vi "Relay Experiment V2 - Curves.vi"() -> ()   [LabVIEW 2020]
uses:
  <vilib>/Analysis/8numeric.llb/1D Numeric Integration.vi
  <vilib>/DAQmx/write.llb/DAQmx Write (Analog 1D Wfm NChan NSamp).vi
  <vilib>/DAQmx/create/channels.llb/DAQmx Create Channel (AO-Voltage-Basic).vi
  <vilib>/DAQmx/configure/timing.llb/DAQmx Timing (Use Waveform).vi
  <vilib>/DAQmx/miscellaneous.llb/DAQmx Fill In Error Info.vi
  <vilib>/Analysis/NI_AALBase.lvlib
  <vilib>/measure/NI_MABase.lvlib
  <vilib>/Analysis/NI_AALPro.lvlib
panel:
  in  "Test Mode?":bool
  out "Charge (mC)":dbl
  in  "Recharge\nAmplitude (mA)":dbl=0.1
  in  "DC-to-AC \nDelay (ms)":dbl
  in  "Pulse\nAmplitude (mA)":dbl=-5.0
  in  "Pulse Plateau\nTime (ms) (g)":dbl=5000.0
  in  "Post-Pulse-\nSecond Curve (j)\nRadius (ms/mA)":dbl=150.0
  in  "Post-Pulse - \nFirst Curve (i)\nRadius (ms/mA)":dbl=50.0
  in  "Post-Pulse Curve \nTotal Time (ms) (h)":dbl=750.0
  in  "Recharge-Pulse -\nSecond Curve (f)\nRadius (ms/mA)":dbl=100.0
  in  "Recharge-Pulse - \nFirst Curve (e)\nRadius (ms/mA)":dbl=2000.0
  in  "Recharge-Pulse Curve\nTotal Time (ms) (d)":dbl=2100.0
  in  "Pre-Recharge -\nSecond Curve (c)\nRadius (ms/mA)":dbl=10000.0
  in  "Pre-Recharge -  \nFirst Curve (b)\nRadius (ms/mA)":dbl=10000.0
  in  "Pre-Recharge\nCurve Total\nTime (ms) (a)":dbl=2000.0
  in  "Trigger 2 Channel":tag="Dev2/ao3"
  in  "AC Output Channel":tag="Dev2/ao1"
  in  "Trigger 1 Channel":tag="Dev2/ao2"
  in  "DC Output Channel":tag="Dev2/ao0"
  in  "Stop":bool
  in  "AC Source\nGain":dbl=5.0
  out "DC On":bool=TRUE
  out "AC On":bool
  in  "Waveform Type":u16(ring) items=["Sine Wave", "Triangle Wave", "Square Wave", "Sawtooth Wave"]
  out "DC Waveform Graph":waveform(dbl)(graph)
  in  "AC  Waveform\nFrequency (Hz)":i32=20000 min=0 max=100000 step=10
  in  "AC  Waveform\nAmplitude\n(Vpp/mApp)":dbl
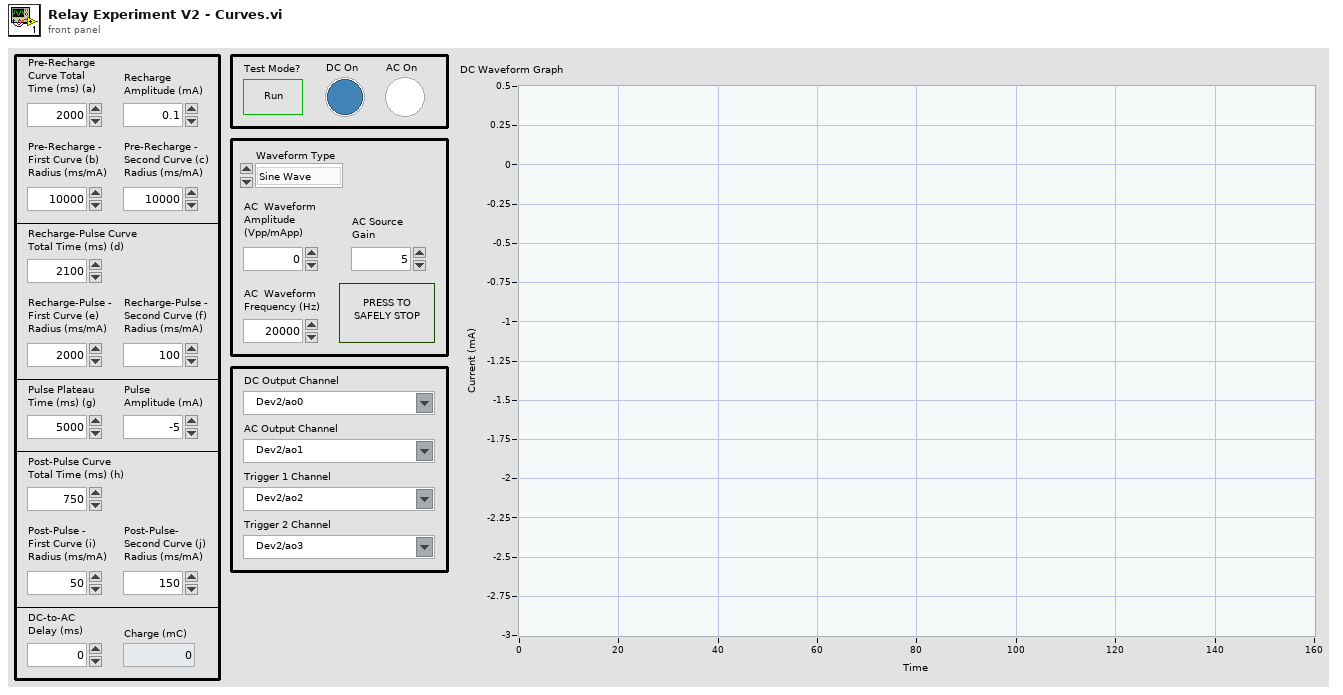
[diagram p1: front panel]
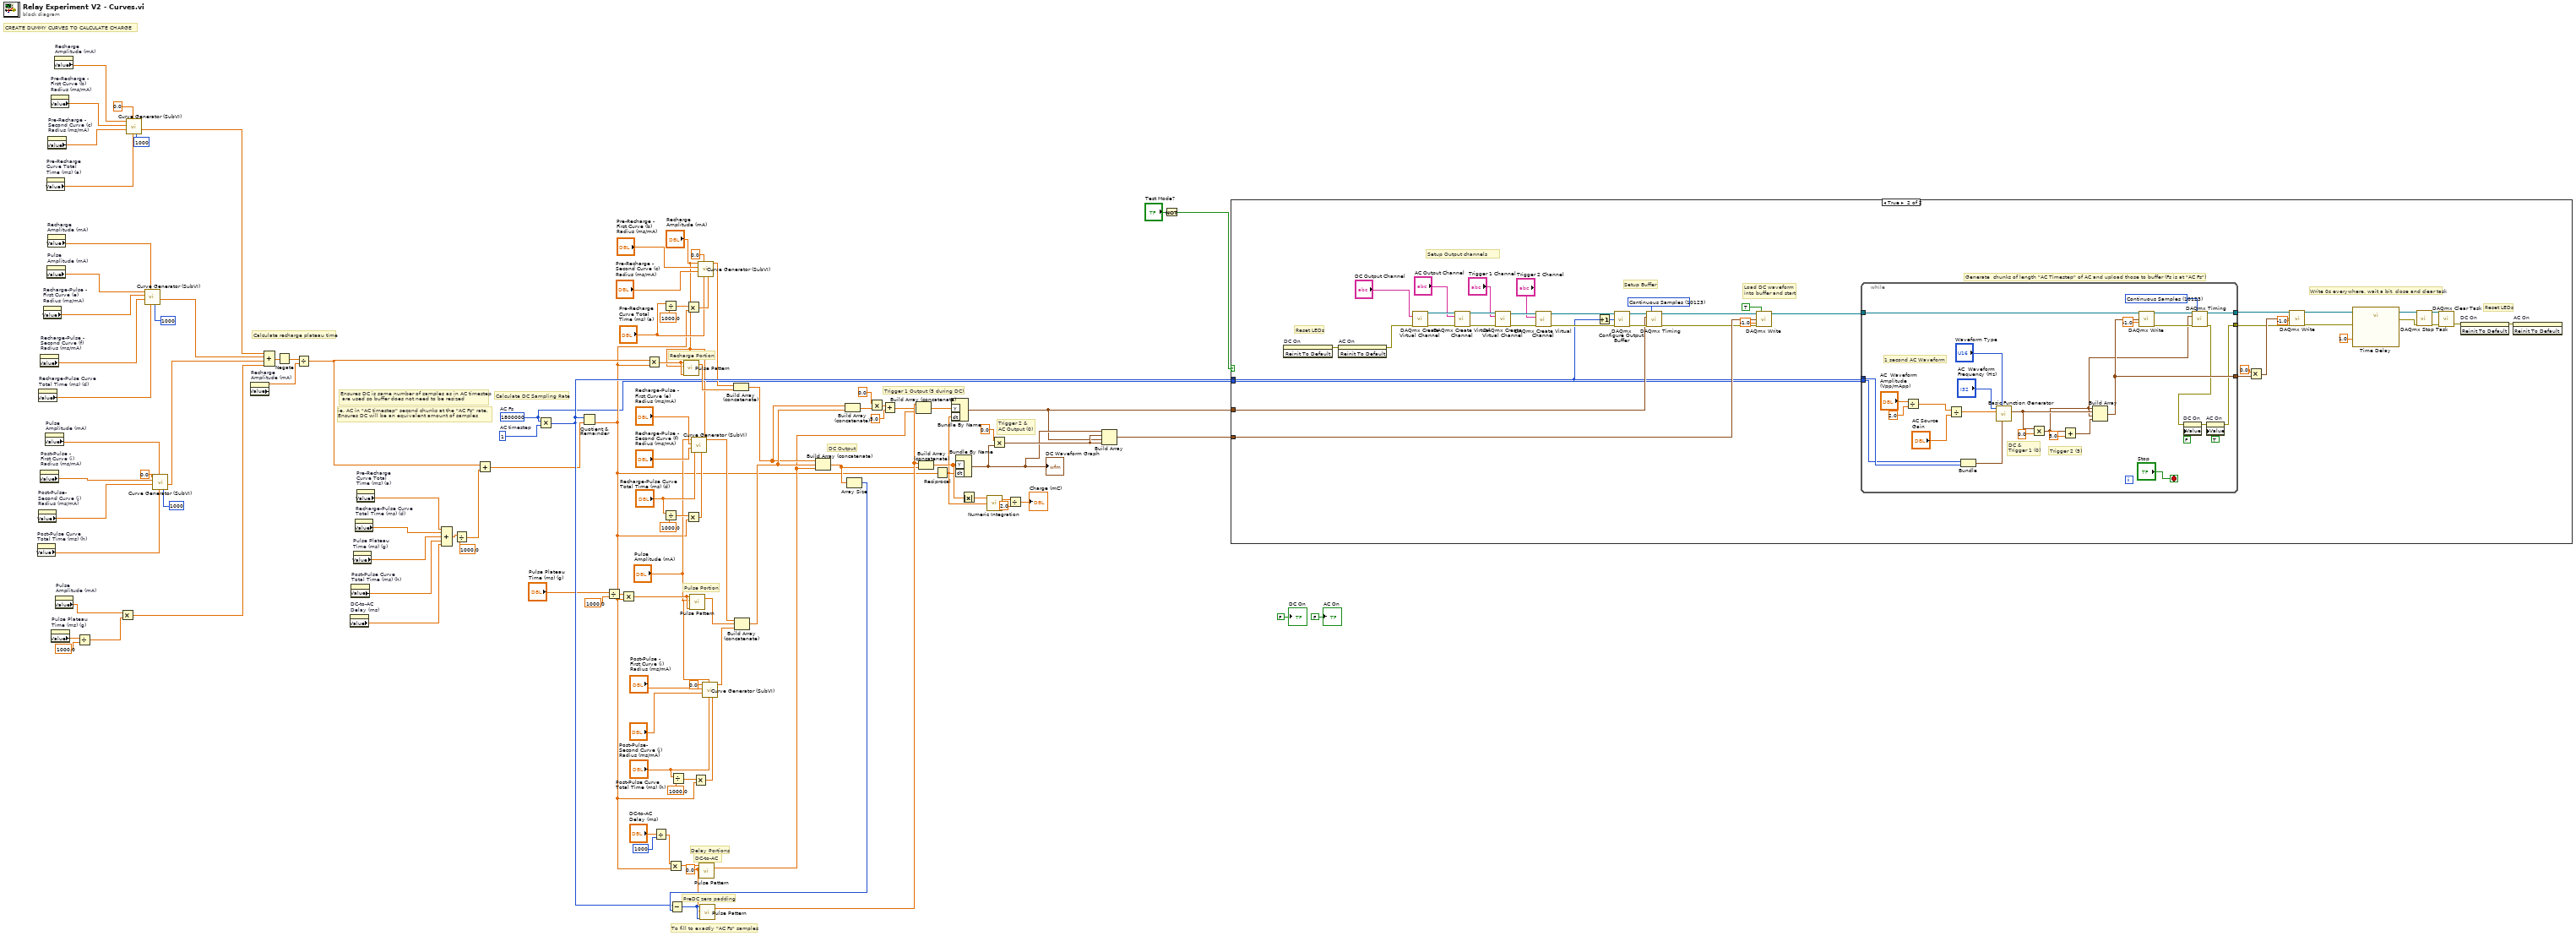
[diagram p0: block diagram]
diagram:
  w82 = 1  # AC timestep
  w8 = 1800000  # AC Fs
  w99 = 0.0 ("amplitude")
  # "Calculate recharge plateau time"
  # "CREATE DUMMY CURVES TO CALCULATE CHARGE"
  # "Trigger 1 Output (5 during DC)"
  # "Trigger 2 &\nAC Output (0)"
  # "DC Output"
  # "ie. AC in \"AC timestep\" second chunks at the \"AC Fs\" rate.  \nEnsures DC will be an equivalent amount of samples"
  # "To fill to exactly \"AC Fs\" samples"
  # "PreDC zero padding"
  # "DC-to-AC"
  # "Ensures DC is same number of samples as in AC timestep\n are used so buffer does not need to be resized"
  # "Calculate DC Sampling Rate"
  # "Delay Portions"
  # "Pulse Portion"
  # "Recharge Portion"
  n1 = property on="Post-Pulse Curve \nTotal Time (ms) (h)" class="DigNum (strict)"() -> ("Value"=w63:dbl)  [unwired: 2 in, 2 out]
  n2 = property on="Post-Pulse-\nSecond Curve (j)\nRadius (ms/mA)" class="DigNum (strict)"() -> ("Value"=w64:dbl)  [unwired: 2 in, 2 out]
  n3 = property on="Recharge-Pulse Curve\nTotal Time (ms) (d)" class="DigNum (strict)"() -> ("Value"=w69:dbl)  [unwired: 2 in, 2 out]
  n4 = property on="Recharge-Pulse -\nSecond Curve (f)\nRadius (ms/mA)" class="DigNum (strict)"() -> ("Value"=w70:dbl)  [unwired: 2 in, 2 out]
  n5 = property on="Post-Pulse - \nFirst Curve (i)\nRadius (ms/mA)" class="DigNum (strict)"() -> ("Value"=w65:dbl)  [unwired: 2 in, 2 out]
  n6 = property on="Recharge-Pulse - \nFirst Curve (e)\nRadius (ms/mA)" class="DigNum (strict)"() -> ("Value"=w71:dbl)  [unwired: 2 in, 2 out]
  n7 = property on="Pulse\nAmplitude (mA)" class="DigNum (strict)"() -> ("Value"=w67:dbl)  [unwired: 2 in, 2 out]
  n8 = property on="Pre-Recharge\nCurve Total\nTime (ms) (a)" class="DigNum (strict)"() -> ("Value"=w72:dbl)  [unwired: 2 in, 2 out]
  n9 = property on="Pulse\nAmplitude (mA)" class="DigNum (strict)"() -> ("Value"=w77:dbl)  [unwired: 2 in, 2 out]
  n10 = property on="Recharge\nAmplitude (mA)" class="DigNum (strict)"() -> ("Value"=w76:dbl)  [unwired: 2 in, 2 out]
  n11 = property on="Pre-Recharge -\nSecond Curve (c)\nRadius (ms/mA)" class="DigNum (strict)"() -> ("Value"=w73:dbl)  [unwired: 2 in, 2 out]
  n12 = property on="Pre-Recharge -  \nFirst Curve (b)\nRadius (ms/mA)" class="DigNum (strict)"() -> ("Value"=w74:dbl)  [unwired: 2 in, 2 out]
  n13 = property on="Pulse Plateau\nTime (ms) (g)" class="DigNum (strict)"() -> ("Value"=w61:dbl)  [unwired: 2 in, 2 out]
  n14 = property on="Recharge\nAmplitude (mA)" class="DigNum (strict)"() -> ("Value"=w80:dbl)  [unwired: 2 in, 2 out]
  n15 = property on="Pulse\nAmplitude (mA)" class="DigNum (strict)"() -> ("Value"=w62:dbl)  [unwired: 2 in, 2 out]
  n16 = Divide(x=w61, y=1000.0) -> (x/y=w59:dbl)
  n17 = Multiply(x=w62, y=w59) -> (x*y=w55:dbl)
  n18 = call "Curve Generator (SubVI).vi"("Number of Samples"=1000, "Total Length (ms)"=w72, "Start Amplitude (mA)"=0.0 ("Start Amplitude"), "Post-ramp\nRadius (ms/mA)"=w73, "Pre-ramp\nRadius (ms/mA)"=w74, "End Amplitude (mA)"=w80) -> ("Charge (mC)"=w58:dbl)  [unwired: 3 in, 2 out]
  n19 = call "Curve Generator (SubVI).vi"("Number of Samples"=1000, "Total Length (ms)"=w69, "Start Amplitude (mA)"=w76, "Post-ramp\nRadius (ms/mA)"=w70, "Pre-ramp\nRadius (ms/mA)"=w71, "End Amplitude (mA)"=w77) -> ("Charge (mC)"=w57:dbl)  [unwired: 3 in, 2 out]
  n20 = call "Curve Generator (SubVI).vi"("Number of Samples"=1000, "Total Length (ms)"=w63, "Start Amplitude (mA)"=w67, "Post-ramp\nRadius (ms/mA)"=w64, "Pre-ramp\nRadius (ms/mA)"=w65, "End Amplitude (mA)"=0.0 ("End Amplitude")) -> ("Charge (mC)"=w56:dbl)  [unwired: 3 in, 2 out]
  n21 = property on="Recharge\nAmplitude (mA)" class="DigNum (strict)"() -> ("Value"=w14:dbl)  [unwired: 2 in, 2 out]
  n22 = Compound Arithmetic op=ADD(w58, w57, w56, w55) -> (w54:dbl)
  n23 = Negate(x=w54) -> (-x=w15:dbl)
  n24 = Divide(x=w15, y=w14) -> (x/y=w53:dbl)
  n25 = property on="DC-to-AC \nDelay (ms)" class="DigNum (strict)"() -> ("Value"=w3:dbl)  [unwired: 2 in, 2 out]
  n26 = property on="Post-Pulse Curve \nTotal Time (ms) (h)" class="DigNum (strict)"() -> ("Value"=w48:dbl)  [unwired: 2 in, 2 out]
  n27 = property on="Pulse Plateau\nTime (ms) (g)" class="DigNum (strict)"() -> ("Value"=w49:dbl)  [unwired: 2 in, 2 out]
  n28 = property on="Recharge-Pulse Curve\nTotal Time (ms) (d)" class="DigNum (strict)"() -> ("Value"=w50:dbl)  [unwired: 2 in, 2 out]
  n29 = property on="Pre-Recharge\nCurve Total\nTime (ms) (a)" class="DigNum (strict)"() -> ("Value"=w52:dbl)  [unwired: 2 in, 2 out]
  n30 = Compound Arithmetic op=ADD(w52, w50, w49, w48, w3) -> (w47:dbl)
  n31 = Divide(x=w47, y=1000.0) -> (x/y=w45:dbl)
  n32 = Add(x=w53, y=w45) -> (x+y=w44:dbl)
  n33 = Multiply(x=w8, y=w82) -> (x*y=w81:i32)
  n34 = Quotient & Remainder(x=w81, y=w44) -> (floor(x/y)=w22:dbl)  [unwired: 1 out]
  n35 = Divide(x="Pulse Plateau\nTime (ms) (g)", y=1000.0) -> (x/y=w18:dbl)
  n36 = Multiply(x=w18, y=w22) -> (x*y=w107:dbl)
  n37 = Multiply(x=w53, y=w22) -> (x*y=w108:dbl)
  n38 = Divide(x="DC-to-AC \nDelay (ms)", y=1000) -> (x/y=w102:dbl)
  n39 = Divide(x="Pre-Recharge\nCurve Total\nTime (ms) (a)", y=1000.0) -> (x/y=w37:dbl)
  n40 = Divide(x="Recharge-Pulse Curve\nTotal Time (ms) (d)", y=1000.0) -> (x/y=w33:dbl)
  n41 = Multiply(x=w102, y=w22) -> (x*y=w104:dbl)
  n42 = Divide(x="Post-Pulse Curve \nTotal Time (ms) (h)", y=1000.0) -> (x/y=w24:dbl)
  n43 = call <vilib>:"Pulse Pattern.vi"("width"=w108, "amplitude"="Recharge\nAmplitude (mA)", "samples"=w108) -> ("Pulse Pattern"=w106:dbl[])  [unwired: 1 in, 1 out]
  n44 = Multiply(x=w37, y=w22) -> (x*y=w40:dbl)
  n45 = Multiply(x=w33, y=w22) -> (x*y=w31:dbl)
  n46 = call <vilib>:"Pulse Pattern.vi"("width"=w107, "amplitude"="Pulse\nAmplitude (mA)", "samples"=w107) -> ("Pulse Pattern"=w105:dbl[])  [unwired: 1 in, 1 out]
  n47 = call "Curve Generator (SubVI).vi"("Number of Samples"=w31, "Total Length (ms)"="Recharge-Pulse Curve\nTotal Time (ms) (d)", "Start Amplitude (mA)"="Recharge\nAmplitude (mA)", "Post-ramp\nRadius (ms/mA)"="Recharge-Pulse -\nSecond Curve (f)\nRadius (ms/mA)", "Pre-ramp\nRadius (ms/mA)"="Recharge-Pulse - \nFirst Curve (e)\nRadius (ms/mA)", "End Amplitude (mA)"="Pulse\nAmplitude (mA)") -> ("S-Curve"=w30:dbl[])  [unwired: 3 in, 2 out]
  n48 = Multiply(x=w24, y=w22) -> (x*y=w21:dbl)
  n49 = call "Curve Generator (SubVI).vi"("Number of Samples"=w40, "Total Length (ms)"="Pre-Recharge\nCurve Total\nTime (ms) (a)", "Start Amplitude (mA)"=0.0, "Post-ramp\nRadius (ms/mA)"="Pre-Recharge -\nSecond Curve (c)\nRadius (ms/mA)", "Pre-ramp\nRadius (ms/mA)"="Pre-Recharge -  \nFirst Curve (b)\nRadius (ms/mA)", "End Amplitude (mA)"="Recharge\nAmplitude (mA)") -> ("S-Curve"=w13:dbl[])  [unwired: 3 in, 2 out]
  n50 = call <vilib>:"Pulse Pattern.vi"("amplitude"=w99, "samples"=w104) -> ("Pulse Pattern"=w90:dbl[])  [unwired: 2 in, 1 out]
  n51 = call "Curve Generator (SubVI).vi"("Number of Samples"=w21, "Total Length (ms)"="Post-Pulse Curve \nTotal Time (ms) (h)", "Start Amplitude (mA)"="Pulse\nAmplitude (mA)", "Post-ramp\nRadius (ms/mA)"="Post-Pulse-\nSecond Curve (j)\nRadius (ms/mA)", "Pre-ramp\nRadius (ms/mA)"="Post-Pulse - \nFirst Curve (i)\nRadius (ms/mA)", "End Amplitude (mA)"=0.0) -> ("S-Curve"=w20:dbl[])  [unwired: 3 in, 2 out]
  n52 = Build Array (concatenate)(w13, w106) -> (w93:dbl[])
  n53 = Build Array (concatenate)(w30, w105, w20) -> (w94:dbl[])
  n54 = Build Array (concatenate)(w93, w94, w90) -> (w83:dbl[])
  n55 = Build Array (concatenate)(w93, w94) -> (w92:dbl[])
  n56 = Array Size(array=w83) -> (size(s)=w101:i32)
  n57 = Subtract(x=w81, y=w101) -> (x-y=w100:i32)
  n58 = call <vilib>:"Pulse Pattern.vi"("width"=w100, "amplitude"=w99, "samples"=w100) -> ("Pulse Pattern"=w91:dbl[])  [unwired: 1 in, 1 out]
  n59 = Multiply(x=0.0 ("amplitude"), y=w92) -> (x*y=w95:dbl[])
  n60 = Add(x=w95, y=5.0) -> (x+y=w86:dbl[])
  n61 = Build Array (concatenate)(w91, w86, w90) -> (w84:dbl[])
  n62 = Build Array (concatenate)(w91, w83) -> (w2:dbl[])
  n63 = Reciprocal(x=w22) -> (1/x=w1:dbl)
  n64 = Bundle By Name("Y"=w84, "dt"=w1) -> (w85:waveform(dbl))  [unwired: 1 in]
  n65 = Bundle By Name("Y"=w2, "dt"=w1) -> (w88:waveform(dbl))  [unwired: 1 in]
  "DC Waveform Graph" <- w88
  n66 = Absolute Value(x=w2) -> (abs(x)=w12:dbl[])
  n67 = call-poly <vilib>:"Numeric Integration.vi"("dt"=w1, "Input Array"=w12) -> ("result"=w11:dbl)  [unwired: 1 in, 1 out]
  n68 = Multiply(x=0.0 ("amplitude"), y=w88) -> (x*y=w89:waveform(dbl))
  n69 = Divide(x=w11, y=2.0) -> (x/y=→"Charge (mC)":dbl)
  n70 = Build Array(w88, w89, w85, w89) -> (w87:waveform(dbl)[])
  n71 = Not(x="Test Mode?") -> (.not. x?=w4:bool)
  n72 = case shown="True" w4 {
    tunnel: w87 -> [_ w134]
    tunnel: w85 -> [_ w111]
    tunnel: w81 -> [_ w110]
    tunnel: w8 -> [_ w109]
    frame False {
    }
    frame True {
      w138 = 10123 items=["Finite Samples"=10178, "Continuous Samples"=10123, "Hardware Timed Single Point"=12522] ("sample mode")
      # "Reset LEDs"
      # "Reset LEDs"
      # "Write 0s everywhere, wait a bit, close and clear task"
      # "Generate  chunks of length \"AC Timestep\" of AC and upload those to buffer (Fs is at \"AC Fs\")"
      # "Load DC waveform\ninto buffer and start"
      # "Setup Buffer"
      # "Setup Output channels"
      n73 = invoke on="DC On" class="Bool (strict)" method="Reinit To Default"() -> (error out=w121:errorcluster)  [unwired: 3 in, 2 out]
      n74 = invoke on="AC On" class="Bool (strict)" method="Reinit To Default"(error in=w121) -> (error out=w120:errorcluster)  [unwired: 2 in, 2 out]
      n75 = call-poly <vilib>:"DAQmx Create Virtual Channel.vi"("physical channels"="DC Output Channel", "error in"=w120) -> ("task out"=w147:refnum<k21>, "error out"=w148:errorcluster)  [unwired: 12 in]
      n76 = call-poly <vilib>:"DAQmx Create Virtual Channel.vi"("task in"=w147, "physical channels"="AC Output Channel", "error in"=w148) -> ("task out"=w144:refnum<k21>, "error out"=w145:errorcluster)  [unwired: 11 in]
      n77 = call-poly <vilib>:"DAQmx Create Virtual Channel.vi"("task in"=w144, "physical channels"="Trigger 1 Channel", "error in"=w145) -> ("task out"=w141:refnum<k21>, "error out"=w142:errorcluster)  [unwired: 11 in]
      n78 = call-poly <vilib>:"DAQmx Create Virtual Channel.vi"("task in"=w141, "physical channels"="Trigger 2 Channel", "error in"=w142) -> ("task out"=w139:refnum<k21>, "error out"=w123:errorcluster)  [unwired: 11 in]
      n79 = Increment(x=w110) -> (x+1=w112:i32)
      n80 = call <vilib>:"DAQmx Configure Output Buffer.vi"("task/channels in"=w139, "buffer size (in samples per channel)"=w112, "error in"=w123) -> ("task out"=w137:refnum<k21>, "error out"=w122:errorcluster)  [unwired: 11 in]
      n81 = call-poly <vilib>:"DAQmx Timing.vi"("task/channels in"=w137, "sample mode"=w138, "waveform"=w111, "error in"=w122) -> ("task out"=w136:refnum<k21>, "error out"=w114:errorcluster)  [unwired: 10 in]
      n82 = call-poly <vilib>:"DAQmx Write.vi"("task/channels in"=w136, "auto start"=TRUE, "data"=w134, "timeout"=-1.0, "error in"=w114) -> ("task out"=w113:refnum<k21>)  [unwired: 8 in, 2 out]
      n83 = while {
        tunnel: w110 -> [w156]
        tunnel: w113 -> [w162]
        tunnel: [w160] -> w131
        tunnel: [w163] -> w132
        tunnel: [w150] -> w117
        tunnel: w109 -> [w155]
        stop <- "Stop" stop-if-true
        w157 = 10123 items=["Finite Samples"=10178, "Continuous Samples"=10123, "Hardware Timed Single Point"=12522] ("sample mode")
        # "1 second AC Waveform"
        # "Trigger 2 (5)"
        # "DC &\nTrigger 1 (0)"
        n84 = Divide(x="AC  Waveform\nAmplitude\n(Vpp/mApp)", y=2.0) -> (x/y=w175:dbl)
        n85 = Divide(x=w175, y="AC Source\nGain") -> (x/y=w173:dbl)
        n86 = Bundle("AC Fs"=w155, w156) -> (w169:cluster{"AC Fs":i32, i32})  [unwired: 1 in]
        n87 = call <vilib>:"Basic Function Generator.vi"("sampling info"=w169, "signal type"="Waveform Type", "amplitude"=w173, "frequency"="AC  Waveform\nFrequency (Hz)") -> ("signal out"=w165:waveform(dbl))  [unwired: 5 in, 2 out]
        n88 = Multiply(x=w165, y=0.0 ("x")) -> (x*y=w158:waveform(dbl))
        n89 = Add(x=w158, y=5.0) -> (x+y=w164:waveform(dbl))
        n90 = Build Array(w158, w165, w158, w164) -> (w163:waveform(dbl)[])
        n91 = call-poly <vilib>:"DAQmx Write.vi"("task/channels in"=w162, "data"=w163, "timeout"=-1.0) -> ("task out"=w159:refnum<k21>, "error out"=w161:errorcluster)  [unwired: 10 in, 1 out]
        n92 = call-poly <vilib>:"DAQmx Timing.vi"("task/channels in"=w159, "sample mode"=w157, "waveform"=w158, "error in"=w161) -> ("task out"=w160:refnum<k21>, "error out"=w151:errorcluster)  [unwired: 10 in]
        n93 = property on="DC On" class="Bool (strict)"(error in=w151, "Value"=FALSE ("DC On")) -> (error out=w154:errorcluster)  [unwired: 1 in, 1 out]
        n94 = property on="AC On" class="Bool (strict)"(error in=w154, "Value"=TRUE ("AC On")) -> (error out=w150:errorcluster)  [unwired: 1 in, 1 out]
      }
      n95 = Multiply(x=0.0, y=w132) -> (x*y=w130:waveform(dbl)[])
      n96 = call-poly <vilib>:"DAQmx Write.vi"("task/channels in"=w131, "data"=w130, "timeout"=-1.0, "error in"=w117) -> ("task out"=w127:refnum<k21>, "error out"=w116:errorcluster)  [unwired: 9 in, 1 out]
      n97 = call "Time Delay"("error in (no error)"=w116, "Delay Time (s)"=1.0) -> ("error out"=w126:errorcluster)  [unwired: 9 in]
      n98 = call <vilib>:"DAQmx Stop Task.vi"("task/channels in"=w127, "error in"=w126) -> ("task out"=w125:refnum<k21>, "error out"=w124:errorcluster)  [unwired: 12 in]
      n99 = call <vilib>:"DAQmx Clear Task.vi"("task in"=w125, "error in"=w124) -> ("error out"=w118:errorcluster)  [unwired: 13 in]
      n100 = invoke on="DC On" class="Bool (strict)" method="Reinit To Default"(error in=w118) -> (error out=w119:errorcluster)  [unwired: 2 in, 2 out]
      n101 = invoke on="AC On" class="Bool (strict)" method="Reinit To Default"(error in=w119) -> ()  [unwired: 2 in, 3 out]
    }
  }
  "AC On" <- FALSE ("AC On")
  "DC On" <- FALSE ("DC On")
